vi "BusIn_read.vi"(8 "error in (no error)":errorcluster, 11 "BusIn in":refnum<class "BusIn.lvclass">) -> (0 "error out":errorcluster, 2 "value":dbl, 3 "BusIn out":refnum<class "BusIn.lvclass">)   [LabVIEW 2011, in "mbed_LVLibrary.lvlib" / "BusIn.lvclass"]
uses:
  BusIn.lvclass
  BusIn.lvclass/BusIn.ctl
  Transport Mechanisms/mbed/mbed.lvclass
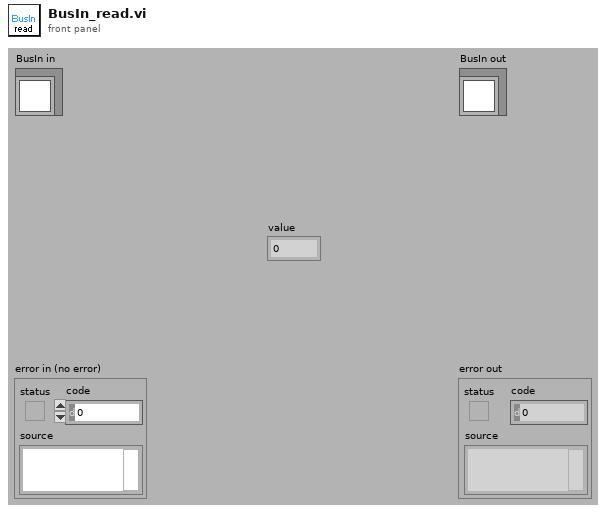
[diagram p1: front panel]
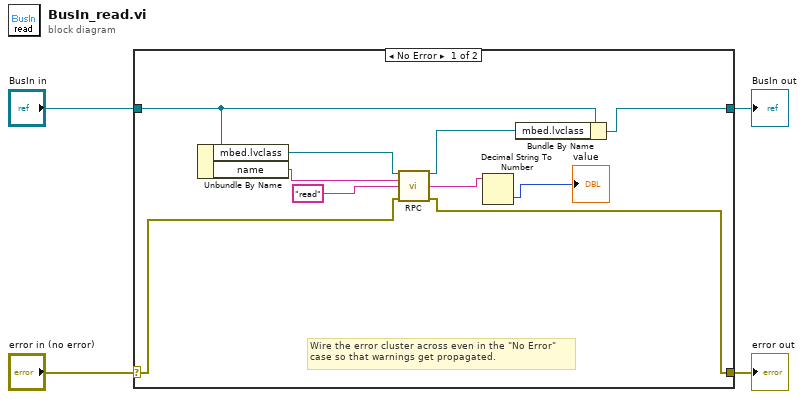
[diagram p0: block diagram]
diagram:
  n1 = case shown="No Error" "error in (no error)" {
    selector: "error in (no error)" -> [w6 w16]
    tunnel: [w5 w16] -> w3
    tunnel: [w9 w15] -> w1
    tunnel: "BusIn in" -> [w8 w15]
    frame No Error {
      # "Wire the error cluster across even in the \"No Error\"\ncase so that warnings get propagated."
      n2 = Unbundle By Name(w8) -> ("mbed.lvclass"=w12:refnum<class "mbed.lvclass">, "name"=w11:string)
      n3 = call-dynamic "RPC.vi"("mbed in"=w12, "Name"=w11, "method"="read", "error in (no error)"=w6) -> ("mbed out"=w7:refnum<class "mbed.lvclass">, "RPC Result"=w13:string, "error out"=w5:errorcluster)  [unwired: 9 in]
      n4 = Decimal String To Number(string=w13) -> (number=→"value":i32)  [unwired: 2 in, 1 out]
      n5 = Bundle By Name(cluster=w8, "mbed.lvclass"=w7) -> (w9:refnum<class "BusIn.lvclass">)
    }
    frame Error {
    }
  }
  "error out" <- w3
  "BusIn out" <- w1
